vi "PH_SHS_Analysis_Statistician.PC Select Data.vi"(0 "i ref in":refnum<vi>, 1 "Stat or Trend":bool, 2 "Data 1":i16, 3 "Data 2":i16, 4 "Data 3":i16, 5 "error in (no error)":errorcluster) -> (14 "i ref out":refnum<vi>, 19 "error out":errorcluster)   [LabVIEW 2014, in "PH_SHS_Analysis_Statistician.lvlib"]
doc: "This VI sets attributes and some GUI elements. It contains the get data to modify / set modified data -vis, handle with care!"
uses:
  PH_SHS_Analysis_Statistician.lvlib
  PH_Basics/PH_Common/PH_Common.lvlib
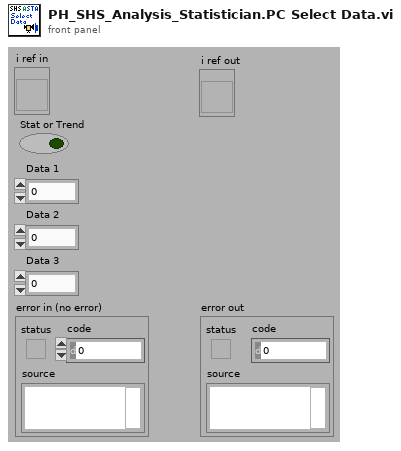
[diagram p1: front panel]
types:
  T1 = typedef "PH_SHS_Analysis_Statistician.lvlib/PH_SHS_Analysis_Statistician.i attribute.ctl" = cluster{"GUI Refs ":cluster{"Status":refnum<vi>, "Result Graph":refnum<vi>, "Mean Data 1":refnum<vi>, "Std Dev Data 1":refnum<vi>, "Mean Data 2":refnum<vi>, "Std Dev Data 2":refnum<vi>, "Mean Data 3":refnum<vi>, "Std Dev Data 3":refnum<vi>, "Dummy Mean":refnum<vi>, "Dummy Std Dev":refnum<vi>, "Export Data":refnum<vi>, "Data 1":refnum<vi>, "Data 2":refnum<vi>, "Data 3":refnum<vi>, "Stat or Trend":refnum<vi>, "Delete":refnum<vi>, "Analyzer":refnum<vi>, "Current Zernike Coefficients":refnum<vi>, "PtV [Lambda]":refnum<vi>, "sample length":refnum<vi>}, "Analyzer":string, "Stat or Trend":bool, "Data 1":i16, "Data 2":i16, "Data 3":i16, "Data":T2[], "sample length":i32, "Datasets strored":i32, "Dataarray Size":i32}
  T2 = typedef "PH_SHS_Analysis.lvlib/PH_SHS_Analysis.Zernike Dataset.ctl" = cluster{"State":T3, "Time Stamp":timestamp, "PtV [lambda]":dbl, "Zernicke Coefficients":T4}
  T3 = typedef "PH_StatusHandler.lvlib/PH_StatusHandler.Status.ctl" = i16
  T4 = typedef "PH_SHS_Analysis.lvlib/PH_SHS_Analysis.Zernike Coefficients.ctl" = cluster{"Tilt x":dbl, "Tilt y":dbl, "Defocus":dbl, "Astig 0°":dbl, "Astig 45°":dbl, "Coma x":dbl, "Coma y":dbl, "Spherical":dbl, "Trefoil 0°":dbl, "Trefoil 30°":dbl, "2nd Astig 0°":dbl, "2nd Astig 45°":dbl, "2nd Coma x":dbl, "2nd Coma y":dbl, "2nd Spherical":dbl}
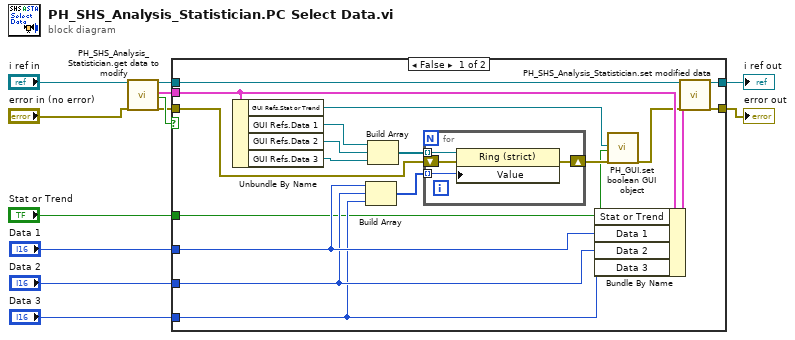
[diagram p0: block diagram]
diagram:
  n1 = call "PH_SHS_Analysis_Statistician.get data to modify.vi"("i ref in"="i ref in", "error in (no error)"="error in (no error)") -> ("i ref out"=w7:refnum<vi>, "i attribute"=w11:T1, "timed out"=w10:bool, "error out"=w6:errorcluster)  [unwired: 14 in]
  n2 = case shown="False" w10 {
    tunnel: w6 -> [w20 w35]
    tunnel: w7 -> [w30 w36]
    tunnel: [w29 w36] -> w8
    tunnel: [w28 w35] -> w9
    tunnel: w11 -> [w26 _]
    tunnel: "Stat or Trend" -> [w13 _]
    tunnel: "Data 1" -> [w19 _]
    tunnel: "Data 2" -> [w18 _]
    tunnel: "Data 3" -> [w17 _]
    frame False {
      n3 = Unbundle By Name(w26) -> ("GUI Refs.Stat or Trend"=w14:refnum<vi>, "GUI Refs.Data 1"=w24:refnum<vi>, "GUI Refs.Data 2"=w23:refnum<vi>, "GUI Refs.Data 3"=w22:refnum<vi>)
      n4 = Build Array(w19, w18, w17) -> (w16:i16[])
      n5 = Build Array(w24, w23, w22) -> (w21:refnum<vi>[])
      n6 = for {
        tunnel: w21 -> [w32] mode=indexing
        shift-right: [w33] -> w25
        shift-left: w20 -> [w34]
        tunnel: w16 -> [w31] mode=indexing
        n7 = property class="Ring (strict)"(reference=w32, error in=w34, "Value"=w31) -> (error out=w33:errorcluster)  [unwired: 1 out]
      }
      n8 = Bundle By Name(cluster=w26, "Stat or Trend"=w13, "Data 1"=w19, "Data 2"=w18, "Data 3"=w17) -> (w27:T1)
      n9 = call "PH_GUI.set boolean GUI object.vi"("Boolean Knob GUI Ref"=w14, "Value"=w13, "error in (no error)"=w25) -> ("error out"=w15:errorcluster)  [unwired: 16 in]
      n10 = call "PH_SHS_Analysis_Statistician.set modified data.vi"("i ref in"=w30, "i attribute"=w27, "error in (no error)"=w15) -> ("i ref out"=w29:refnum<vi>, "error out"=w28:errorcluster)  [unwired: 15 in]
    }
    frame True {
    }
  }
  "error out" <- w9
  "i ref out" <- w8
